vi "generate image series filename.vi"(5 "frame number in":i32, 7 "no..of.frames.to.acquire":dbl, 8 "channel":dbl=-1.0, 11 "Path IN":path) -> (3 "appended path":path)   [LabVIEW 2012]
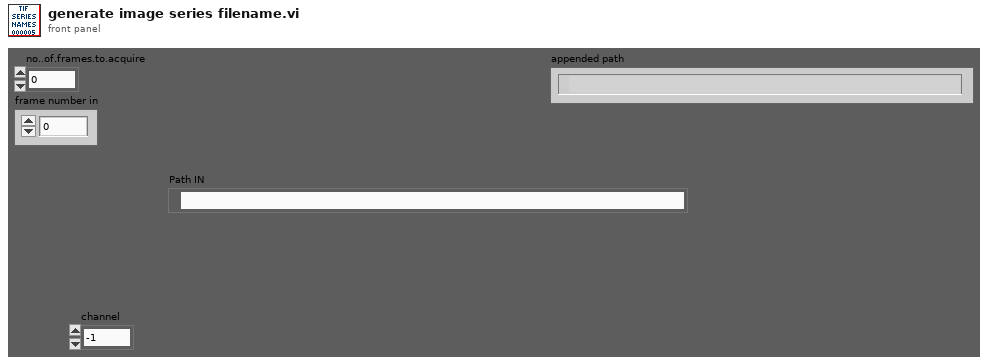
[diagram p1: front panel]
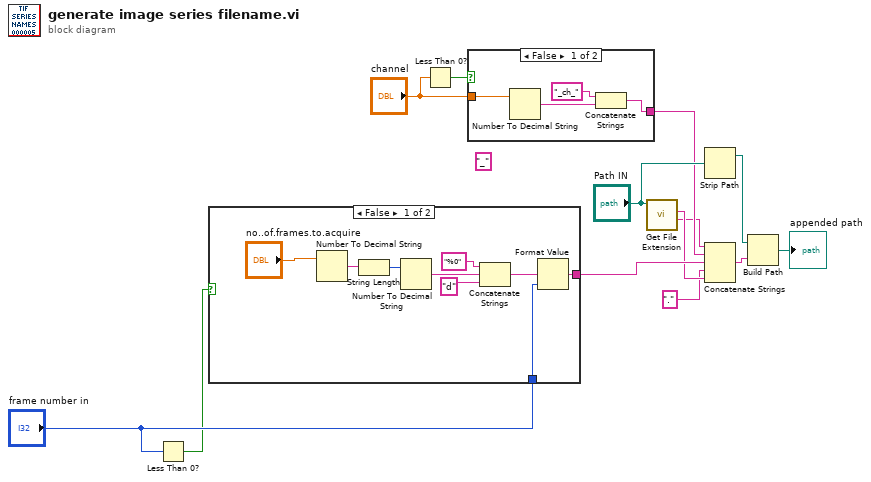
[diagram p0: block diagram]
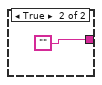
[diagram p2: hidden frame]
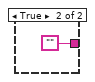
[diagram p3: hidden frame]
diagram:
  (unwired) "_" ("string")
  n1 = Less Than 0?(x="frame number in") -> (x < 0?=w3:bool)
  n2 = case shown="False" w3 {
    tunnel: [w15 ""] -> w12
    tunnel: "frame number in" -> [w14 _]
    frame False {
      n3 = Number To Decimal String(number="no..of.frames.to.acquire") -> (decimal integer string=w21:string)  [unwired: 1 in]
      n4 = String Length(string=w21) -> (length=w20:i32)
      n5 = Number To Decimal String(number=w20) -> (decimal integer string=w19:string)  [unwired: 1 in]
      n6 = Concatenate Strings("%0" ("string"), w19, "d" ("string")) -> (w16:string)
      n7 = Format Value(format string=w16, value (0)=w14) -> (output string=w15:string)  [unwired: 1 in]
    }
    frame True {
    }
  }
  n8 = Less Than 0?(x="channel") -> (x < 0?=w8:bool)
  n9 = case shown="False" w8 {
    tunnel: [w24 ""] -> w2
    tunnel: "channel" -> [w27 _]
    frame False {
      n10 = Number To Decimal String(number=w27) -> (decimal integer string=w25:string)  [unwired: 1 in]
      n11 = Concatenate Strings("_ch_" ("string"), w25) -> (w24:string)
    }
    frame True {
    }
  }
  n12 = call <vilib>:"Get File Extension.vi"("file"="Path IN") -> ("filename without extension"=w1:string, "lowercase file extension"=w6:string)  [unwired: 7 in, 2 out]
  n13 = Strip Path(path="Path IN") -> (stripped path=w10:path)  [unwired: 1 out]
  n14 = Concatenate Strings(w1, w2, w12, "." ("string"), w6) -> (w11:string)
  n15 = Build Path(base path=w10, name or relative path=w11) -> (appended path=→"appended path":path)
